vi "Get Destination Name.vi"(8 "error in (no error)":errorcluster, 10 "Default Destinations":T1, 11 "EXE in":refnum<class "NI_AB_API_EXE.lvclass">) -> (0 "error out":errorcluster, 2 "Destination Name":string, 3 "EXE out":refnum<class "NI_AB_API_EXE.lvclass">)   [LabVIEW 2020, in "NI_AB_API_EXE.lvclass"]
uses:
  <vilib>/AppBuilder/AB_API/EXE/NI_AB_API_EXE.lvclass
  <vilib>/AppBuilder/AB_API/common/AB_API Default Destinations.ctl
  <vilib>/AppBuilder/AB_API/Application/NI_AB_API_Application.lvclass
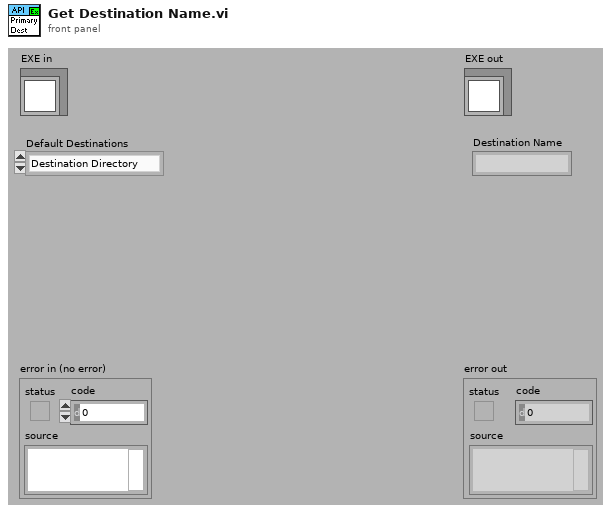
[diagram p1: front panel]
types:
  T1 = typedef "AB_API Default Destinations.ctl" = enum16{"Destination Directory", "Support Directory"}
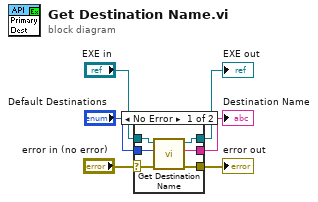
[diagram p0: block diagram]
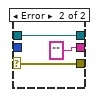
[diagram p2: hidden frame]
diagram:
  n1 = case shown="No Error" "error in (no error)" {
    selector: "error in (no error)" -> [w7 w14]
    tunnel: [w8 w14] -> w5
    tunnel: [w11 w15] -> w3
    tunnel: "EXE in" -> [w12 w15]
    tunnel: [w9 "" ("Destination Name")] -> w2
    tunnel: "Default Destinations" -> [w10 _]
    frame No Error {
      n2 = call-parent "Get Destination Name.vi"("error in (no error)"=w7, "Default Destinations"=w10, "NI_AB_API_Build in"=w12) -> ("error out"=w8:errorcluster, "Destination Name"=w9:string, "NI_AB_API_Build out"=w11:refnum<class "NI_AB_API_EXE.lvclass">)  [unwired: 6 in]
    }
    frame Error {
    }
  }
  "error out" <- w5
  "EXE out" <- w3
  "Destination Name" <- w2
